vi "FABR-Restore Defaults.vi"() -> (4 "Params":T1={"Stimulus"={"Ear"=enum."Left", "Start (kHz)"=0.0, "Stop (kHz)"=16.0, "Step (oct)"=5.0, "Start (dB)"=0, "Stop (dB)"=30, "Step (dB)"=5, "Rep rate (/sec)"=30.0, "Alternate Polarity"=FALSE, "Skip (oct)"=0.0}, "Response"={"Gain"=1.0, "Averages"=0, "Window (ms)"=0.0}, "Hidden"={"AI Samp Rate Hz"=10000.0, "AO Samp Rate Hz"=512.0, "Duration (ms)"=8.5, "Ramp (ms)"=8.5, "Frame size (s)"=0.0}, "Reject"=0.0} {"Response"."Window (ms)" format="%.2f"; "Stimulus"."Start (kHz)" step=5.0; "Stimulus"."Start (dB)" step=5}, 8 "Threshold Estimation":T5={"Tmin (ms)"=1.0, "Tmax (ms)"=6.0, "CC criterion"=0.35, "adjR2 criterion"=0.7}, 15 "error out":errorcluster)   [LabVIEW 2020]
uses:
  Typedefs/FABR-Parameters.ctl
  Typedefs/FABR-Stimulus.ctl
  Typedefs/FABR-Response.ctl
  Typedefs/FABR-Hidden Params.ctl
  Threshold Estimation VIs/ABR3-Threshold Estimation Parameters.ctl
panel:
  in  "Default":T1={"Stimulus"={"Ear"=enum."Right", "Start (kHz)"=4.0, "Stop (kHz)"=32.0, "Step (oct)"=0.5, "Start (dB)"=0, "Stop (dB)"=80, "Step (dB)"=5, "Rep rate (/sec)"=30.0, "Alternate Polarity"=FALSE, "Skip (oct)"=1.0}, "Response"={"Gain"=10000.0, "Averages"=512, "Window (ms)"=8.5}, "Hidden"={"AI Samp Rate Hz"=25000.0, "AO Samp Rate Hz"=100000.0, "Duration (ms)"=5.0, "Ramp (ms)"=0.5, "Frame size (s)"=1.0}, "Reject"=15.0} {"Response"."Window (ms)" format="%.2f"; "Stimulus"."Start (kHz)" step=5.0; "Stimulus"."Start (dB)" step=5}
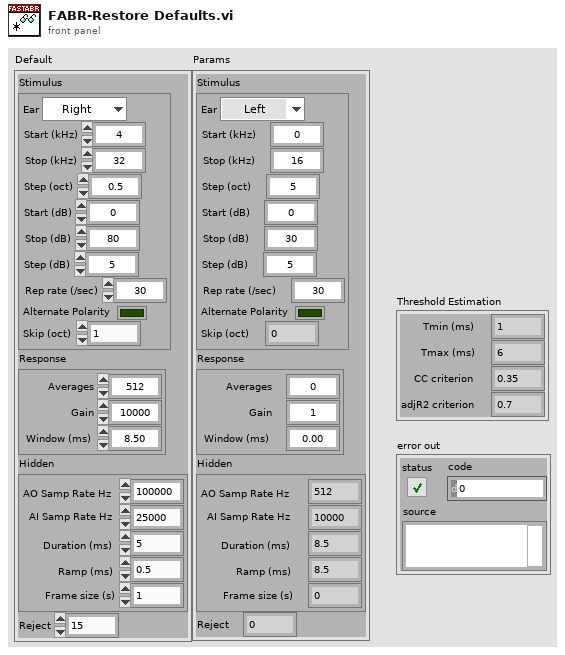
[diagram p1: front panel]
types:
  T1 = typedef "FABR-Parameters.ctl" = cluster{"Stimulus":T2, "Response":T3, "Hidden":T4, "Reject":dbl}
  T2 = typedef "FABR-Stimulus.ctl" = cluster{"Ear":enum16{"Right", "Left"}, "Start (kHz)":dbl, "Stop (kHz)":dbl, "Step (oct)":dbl, "Start (dB)":i32, "Stop (dB)":i32, "Step (dB)":i32, "Rep rate (/sec)":dbl, "Alternate Polarity":bool, "Skip (oct)":dbl}
  T3 = typedef "FABR-Response.ctl" = cluster{"Gain":dbl, "Averages":i32, "Window (ms)":sgl}
  T4 = typedef "FABR-Hidden Params.ctl" = cluster{"AI Samp Rate Hz":dbl, "AO Samp Rate Hz":dbl, "Duration (ms)":dbl, "Ramp (ms)":dbl, "Frame size (s)":dbl}
  T5 = typedef "ABR3-Threshold Estimation Parameters.ctl" = cluster{"Tmin (ms)":dbl, "Tmax (ms)":dbl, "CC criterion":dbl, "adjR2 criterion":dbl}
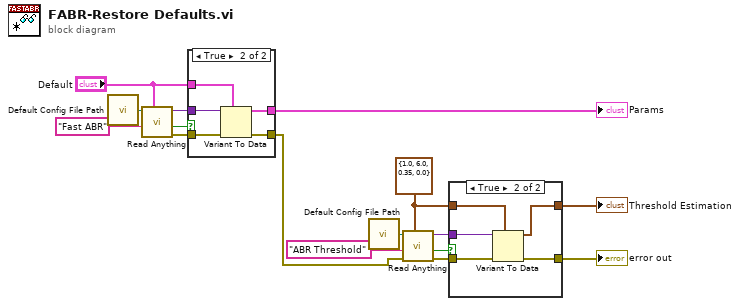
[diagram p0: block diagram]
diagram:
  w9 = T5 {"Tmin (ms)"=1.0, "Tmax (ms)"=6.0, "CC criterion"=0.35, "adjR2 criterion"=0.0} ("Threshold Estimation")
  n1 = call "Default Config File Path.vi"() -> ("Default config file name"=w15:path)
  n2 = call "Read Anything.vi"("Type of Anything"="Default", "Section Name (Name of \"Type of Anything\")"="Fast ABR" ("Section Name (Name of \"Type of Anything\")"), "Path (dialog)"=w15) -> ("Error Out"=w13:errorcluster, "Found?"=w1:bool, "Anything"=w16:variant)  [unwired: 6 in]
  n3 = case shown="True" w1 {
    tunnel: w16 -> [_ w23]
    tunnel: w13 -> [w17 w22]
    tunnel: [w18 w21] -> w12
    tunnel: [w17 w20] -> w6
    tunnel: "Default" -> [w18 w19]
    frame False {
    }
    frame True {
      n4 = Variant To Data(error in=w22, type=w19, Variant=w23) -> (data=w21:T1, error out=w20:errorcluster)
    }
  }
  "Params" <- w12
  n5 = call "Default Config File Path.vi"() -> ("Default config file name"=w8:path)
  n6 = call "Read Anything.vi"("Type of Anything"=w9, "Error In"=w6, "Section Name (Name of \"Type of Anything\")"="ABR Threshold" ("Section Name (Name of \"Type of Anything\")"), "Path (dialog)"=w8) -> ("Error Out"=w3:errorcluster, "Found?"=w5:bool, "Anything"=w4:variant)  [unwired: 5 in]
  n7 = case shown="True" w5 {
    tunnel: w4 -> [_ w29]
    tunnel: w9 -> [w25 w28]
    tunnel: w3 -> [w24 w30]
    tunnel: [w25 w27] -> w10
    tunnel: [w24 w26] -> w11
    frame False {
    }
    frame True {
      n8 = Variant To Data(error in=w30, type=w28, Variant=w29) -> (data=w27:T5, error out=w26:errorcluster)
    }
  }
  "error out" <- w11
  "Threshold Estimation" <- w10
